vi "get terminal info.vi"(8 "error in (no error)":errorcluster, 10 "Get Object Terminals Argument":T2, 11 "Data Cluster in":T1) -> (0 "error out":errorcluster, 2 "String":string, 3 "Data Cluster out":T1)   [LabVIEW 2025, in "Scripting Server.lvlib"]
uses:
  Scripting Server.lvlib
  Module Data--cluster.ctl
  Get Object Terminals Argument--cluster.ctl
  Get Object Terminals (Reply Payload)--cluster.ctl
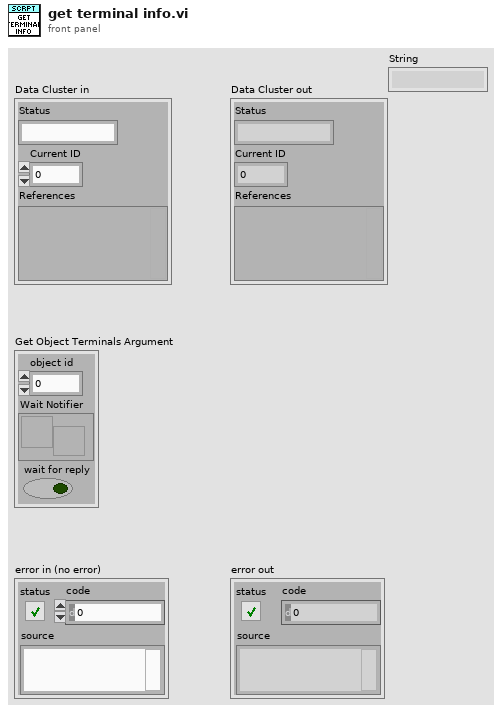
[diagram p1: front panel]
types:
  T1 = typedef "Scripting Server.lvlib/Module Data--cluster.ctl" = cluster{"Status":string, "Current ID":i32, "References":variant}
  T2 = typedef "Scripting Server.lvlib/Get Object Terminals Argument--cluster.ctl" = cluster{"object id":i32, "Wait Notifier":refnum<notifier>, "wait for reply":bool}
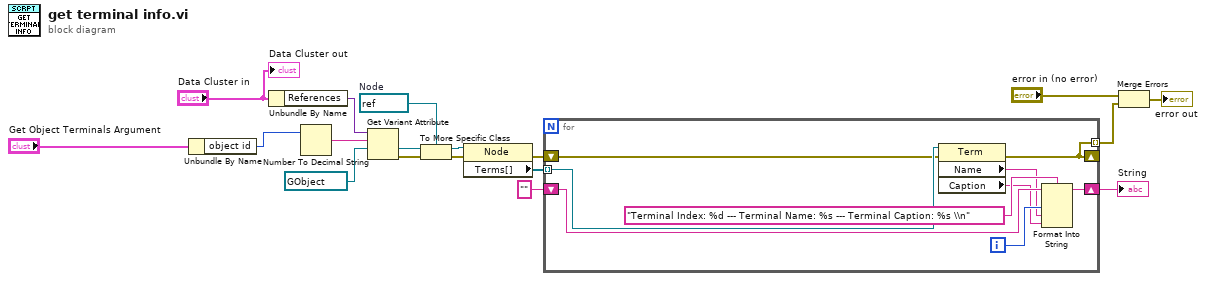
[diagram p0: block diagram]
diagram:
  w6 = refnum<vi> refnum  # Node
  n1 = Unbundle By Name("Get Object Terminals Argument") -> ("object id"=w13:i32)
  n2 = Unbundle By Name("Data Cluster in") -> ("References"=w14:variant)
  n3 = Number To Decimal String(number=w13) -> (decimal integer string=w12:string)  [unwired: 1 in]
  n4 = Get Variant Attribute(Variant=w14, name=w12, default value (empty Variant)=refnum<vi> refnum ("reference")) -> (value=w8:refnum<vi>, error out=w10:errorcluster)  [unwired: 1 in, 2 out]
  n5 = To More Specific Class(target class=w6, reference=w8, error in=w10) -> (specific class reference=w7:refnum<vi>, error out=w9:errorcluster)
  n6 = property class="Node"(reference=w7, error in=w9) -> (error out=w3:errorcluster, "Terms[]"=w4:refnum<vi>[])  [unwired: 1 out]
  n7 = for {
    shift-right: [w26] -> w2
    shift-left: "" -> [w27]
    tunnel: w4 -> [w23] mode=indexing
    shift-right: [w19] -> _
    shift-left: w3 -> [w22]
    tunnel: [w19] -> w1 mode=indexing
    i -> [w24]
    n8 = property class="Term"(reference=w23, error in=w22) -> (error out=w19:errorcluster, "Name"=w21:string, "Caption"=w20:string)  [unwired: 1 out]
    n9 = Format Into String(format string="Terminal Index: %d --- Terminal Name: %s --- Terminal Caption: %s \\n", initial string=w27, w24, w21, w20) -> (resulting string=w26:string)  [unwired: 1 in, 1 out]
  }
  "String" <- w2
  n10 = Merge Errors("error in (no error)", w1) -> (→"error out":errorcluster)
  "Data Cluster out" <- "Data Cluster in"
